vi "Motion Done.vi"(8 "error in (no error)":errorcluster, 10 "Axis":i32, 11 "Simulated-TS in":refnum<class "Simulated-TS.lvclass">) -> (0 "error out":errorcluster, 2 "Done":bool, 3 "Simulated-TS out":refnum<class "Simulated-TS.lvclass">)   [LabVIEW 2019, in "Simulated-TS.lvclass"]
uses:
  Simulated-TS.lvclass
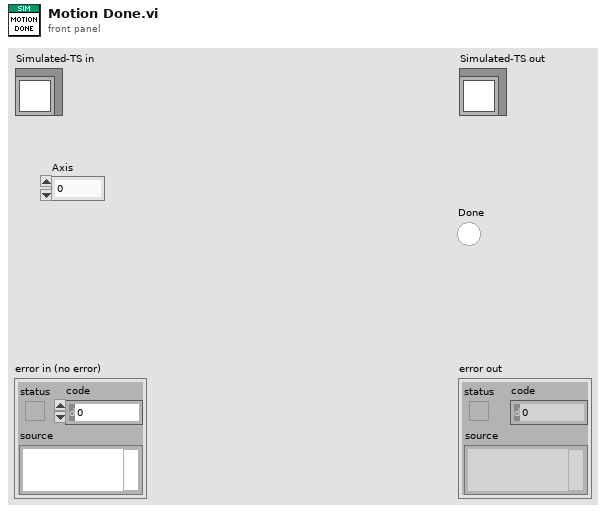
[diagram p1: front panel]
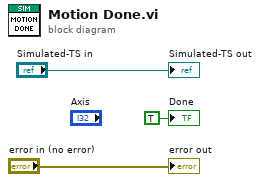
[diagram p0: block diagram]
diagram:
  "error out" <- "error in (no error)"
  "Simulated-TS out" <- "Simulated-TS in"
  "Done" <- TRUE ("Done")
